vi "rm.server.get waveform inputs.vi"(8 "error in (no error)":errorcluster, 11 "Item Ref in":T1 format="%.0x") -> (0 "error out":errorcluster, 3 "Item Ref out":T1 format="%.0x")   [LabVIEW 2016, in "RM.Server.lvlib"]
uses:
  <vilib>/NI Veristand/Custom Device API/Custom Device Item Ref.ctl
  RM.Server.lvlib
  <vilib>/NI VeriStand/Custom Device API/Custom Device API.lvlib
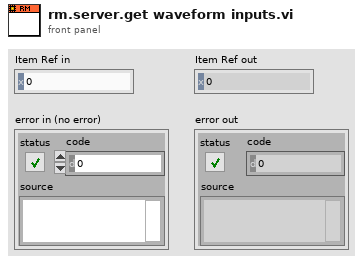
[diagram p1: front panel]
types:
  T1 = typedef "Custom Device API.lvlib/Custom Device Item Ref.ctl" = u64
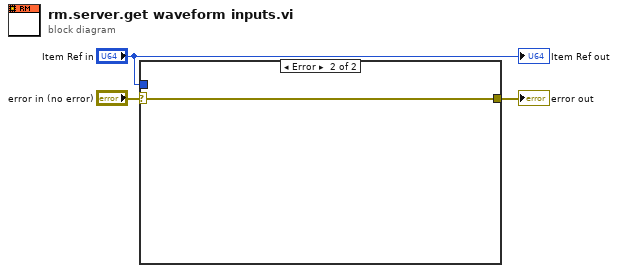
[diagram p0: block diagram]
diagram:
  n1 = case shown="Error" "error in (no error)" {
    selector: "error in (no error)" -> [w4 w5]
    tunnel: [w4 w5] -> w2
    tunnel: "Item Ref in" -> [_ _]
    frame No Error {
    }
    frame Error {
    }
  }
  "error out" <- w2
  "Item Ref out" <- "Item Ref in"
